vi "DataLib.application example read data file.vi"() -> ()   [LabVIEW 2014, in "DataLib.lvlib"]
doc: "This routine demonstrates how to unpack data from a file written with the DiscArchiver. This routine is \"quick and dirty\" to demonstrate the principle."
uses:
  DataLib.lvlib
  CSCore/BaseProcess/BaseProcess.descriptor string definition.ctl
  CSCore/CSSystem/CoreDefs/CoreDefs.rawDataType.ctl
  CSCore/CSSystem/CoreLib/CoreLib.byte array 2 string.vi
  CSCore/CSSystem/CoreLib/CoreLib.byte array 2 double.vi
  CSCore/CSSystem/CoreLib/CoreLib.byte array 2 double array.vi
  CSCore/CSSystem/CoreLib/CoreLib.lvlib
  CSCore/BaseProcess/BaseProcess.lvlib
panel:
  out "subEventData (assuming waveform)":waveform(dbl)[](array[waveform])
  out "subEventDataDisplay (assuming waveform)":waveform(dbl)[](graph)
  out "eventTimestamps":timestamp[](array[timestamp])
  out "headerIDs":timestamp[](array[timestamp])
  out "fileName":path
  out "headerID":timestamp
  out "subeventData":string[][](array[string])
  out "dataDescriptors":T1[][](array[typedef])
  out "daqObjects":string[][](array[string])
  out "eventIDs":i32[](array[numeric])
  out "DaqDevs":string[](array[string])
  out "header":string
  out "dataLength":i32
  # "fileInfo"
  # "dataDescription (header)"
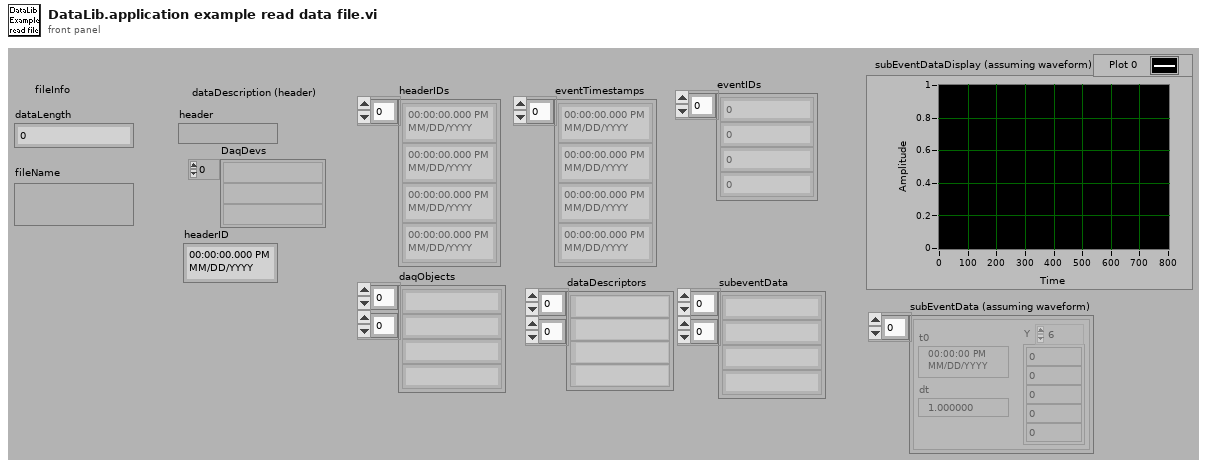
[diagram p1: front panel]
types:
  T1 = typedef "BaseProcess.lvlib/BaseProcess.descriptor string definition.ctl" = string
  T2 = typedef "CoreDefs.rawDataType.ctl" = i8[]
  T3 = enum16{"open", "open or create", "create or replace", "create", "open (read only)"}
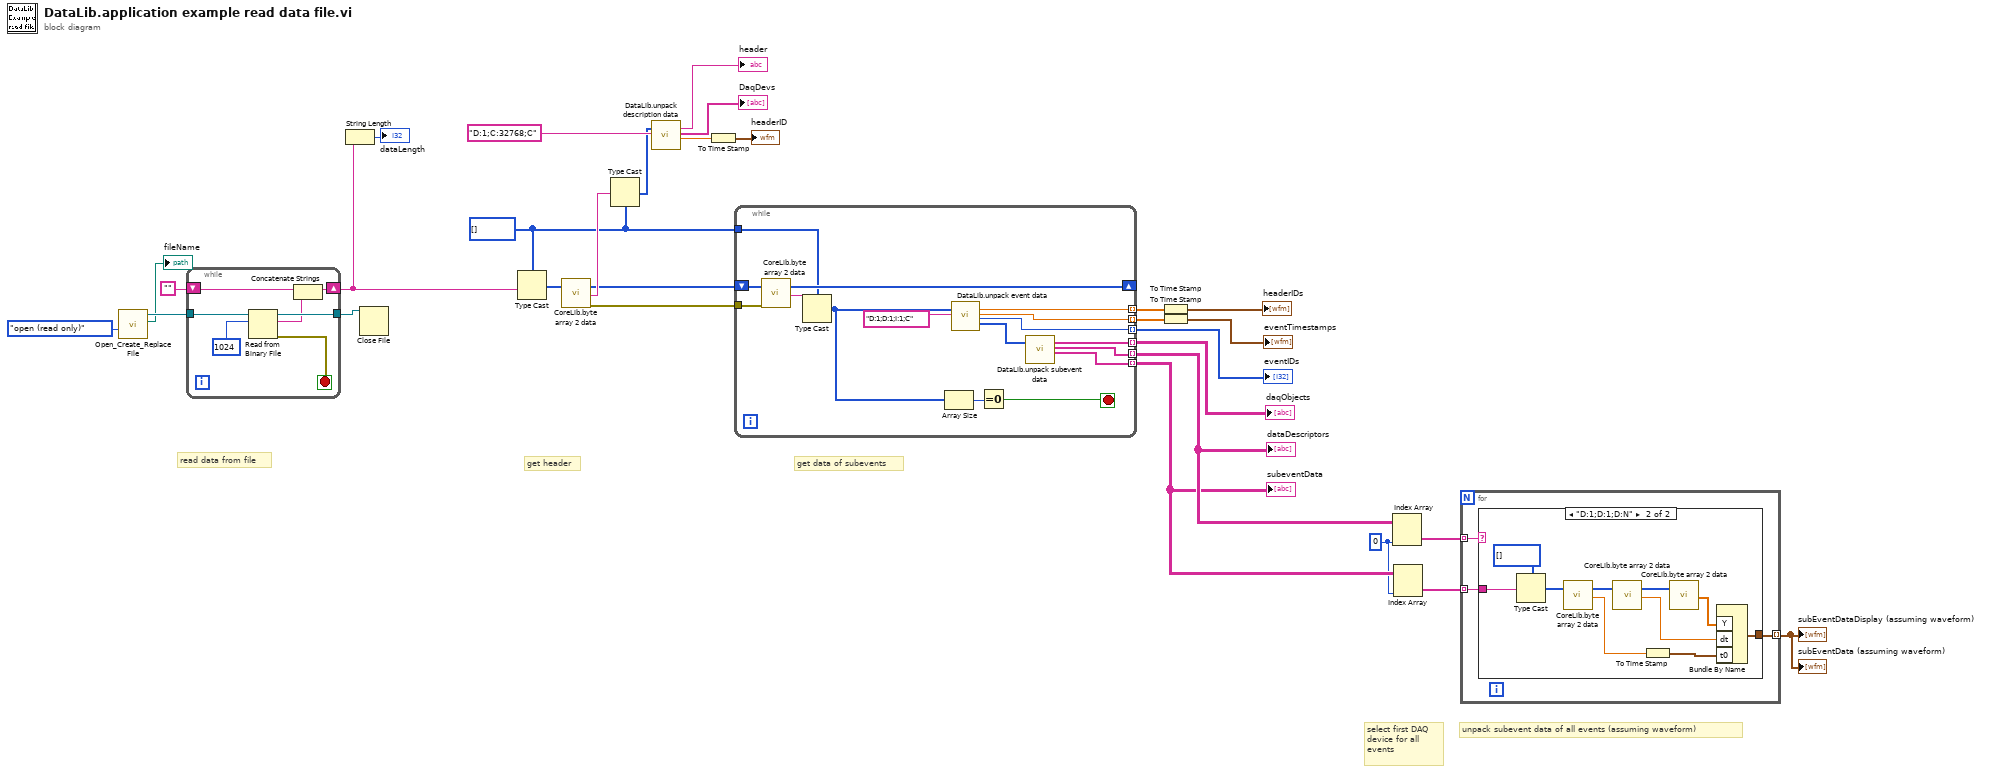
[diagram p0: block diagram]
diagram:
  w1 = 0 ("index (row)")
  w15 = T2 [] ("byteArray")
  # "unpack subevent data of all events (assuming waveform)"
  # "select first DAQ\ndevice for all\nevents"
  # "get data of subevents"
  # "get header"
  # "read data from file"
  n1 = call <vilib>:"Open_Create_Replace File.vi"("function (open:0)"=T3."open (read only)") -> ("new file path"=→"fileName":path, "refnum"=w29:refnum<file>)  [unwired: 7 in, 2 out]
  n2 = while "read data from file" {
    tunnel: w29 -> [w37]
    tunnel: [w36] -> w27
    shift-right: [w31] -> w25
    shift-left: "" -> [w34]
    stop <- w32 stop-if-true
    n3 = Read from Binary File(10:1024 ("count"), 11:w37) -> (0:w32:errorcluster, 2:w33:string, 3:w36:refnum<file>)  [unwired: 4 in, 1 out]
    n4 = Concatenate Strings(w34, w33) -> (w31:string)
  }
  n5 = String Length(string=w25) -> (length=→"dataLength":i32)
  n6 = Close File(refnum=w27) -> ()  [unwired: 1 in, 2 out]
  n7 = Type Cast(type=w15, x=w25) -> (*(type *) &x=w24:T2)
  n8 = call-poly "CoreLib.byte array 2 data.vi"("byteArray"=w24) -> ("byteArray out"=w17:T2, "string"=w18:string, "error out"=w16:errorcluster)  [unwired: 16 in]
  n9 = Type Cast(type=w15, x=w18) -> (*(type *) &x=w19:T2)
  n10 = call "DataLib.unpack description data.vi"("serviceData"=w19, "descriptor"="D:1;C:32768;C") -> ("header"=→"header":string, "DaqDevs"=→"DaqDevs":string[], "headerID"=w20:dbl)  [unwired: 14 in, 1 out]
  n11 = To Time Stamp(1:w20) -> (0:→"headerID":timestamp)
  n12 = while {
    tunnel: w16 -> [w52]
    shift-right: [w50] -> _
    shift-left: w17 -> [w53]
    tunnel: w15 -> [w48]
    tunnel: [w45] -> w14 mode=indexing
    tunnel: [w44] -> w13 mode=indexing
    tunnel: [w43] -> w12 mode=indexing
    tunnel: [w41] -> w11 mode=indexing
    tunnel: [w40] -> w6 mode=indexing
    tunnel: [w39] -> w5 mode=indexing
    stop <- w51 stop-if-true
    n13 = call-poly "CoreLib.byte array 2 data.vi"("byteArray"=w53, "error in (no error)"=w52) -> ("byteArray out"=w50:T2, "string"=w49:string)  [unwired: 15 in, 1 out]
    n14 = Type Cast(type=w48, x=w49) -> (*(type *) &x=w46:T2)
    n15 = Array Size(array=w46) -> (size(s)=w47:i32)
    n16 = call "DataLib.unpack event data.vi"("serviceData"=w46, "descriptor"="D:1;D:1;I:1;C") -> ("headerID"=w45:dbl, "timestamp"=w44:dbl, "eventID"=w43:i32, "subEventData"=w42:T2)  [unwired: 13 in, 1 out]
    n17 = Equal To 0?(x=w47) -> (x = 0?=w51:bool)
    n18 = call "DataLib.unpack subevent data.vi"("subeventData"=w42) -> ("daqObjects"=w41:string[], "dataDescriptors"=w40:T1[], "subeventData"=w39:string[])  [unwired: 15 in, 1 out]
  }
  "eventIDs" <- w12
  "daqObjects" <- w11
  "dataDescriptors" <- w6
  "subeventData" <- w5
  n19 = To Time Stamp(1:w14) -> (0:→"headerIDs":timestamp[])
  n20 = To Time Stamp(1:w13) -> (0:→"eventTimestamps":timestamp[])
  n21 = Index Array(array=w6, index (col)=w1) -> (element=w4:T1[])  [unwired: 1 in]
  n22 = Index Array(array=w5, index (col)=w1) -> (element=w3:string[])  [unwired: 1 in]
  n23 = for {
    tunnel: w4 -> [w56] mode=indexing
    tunnel: w3 -> [w55] mode=indexing
    tunnel: [w54] -> w2 mode=indexing
    n24 = case shown="\"D:1;D:1;D:N\"" w56 {
      tunnel: w55 -> [_ w66]
      tunnel: [_ w57] -> w54
      frame "False", Default {
      }
      frame "D:1;D:1;D:N" {
        n25 = Type Cast(type=T2 [] ("Array"), x=w66) -> (*(type *) &x=w65:T2)
        n26 = call-poly "CoreLib.byte array 2 data.vi"("byteArray"=w65) -> ("byteArray out"=w63:T2, "d64"=w61:dbl)  [unwired: 16 in, 1 out]
        n27 = call-poly "CoreLib.byte array 2 data.vi"("byteArray"=w63) -> ("byteArray out"=w62:T2, "d64"=w58:dbl)  [unwired: 16 in, 1 out]
        n28 = To Time Stamp(1:w61) -> (0:w59:timestamp)
        n29 = call-poly "CoreLib.byte array 2 data.vi"("byteArray"=w62) -> ("[d64]"=w60:dbl[])  [unwired: 16 in, 2 out]
        n30 = Bundle By Name("Y"=w60, "dt"=w58, "t0"=w59) -> (w57:waveform(dbl))  [unwired: 1 in]
      }
    }
  }
  "subEventDataDisplay (assuming waveform)" <- w2
  "subEventData (assuming waveform)" <- w2
